vi "Read Path Connection Map.vi"(8 "error in (no error)":errorcluster, 11 "Cal Standard Base in":refnum<class "Cal Standard Base.lvclass">) -> (0 "error out":errorcluster, 2 "Path Connection Map":map{string, string[]}(c390), 3 "Cal Standard Base out":refnum<class "Cal Standard Base.lvclass">)   [LabVIEW 2023, in "RFFixtureCharact.Instruments.lvlib" / "Cal Standard Base.lvclass"]
uses:
  Cal Standard Base.lvclass
  Cal Standard Base.lvclass/Cal Standard Base.ctl
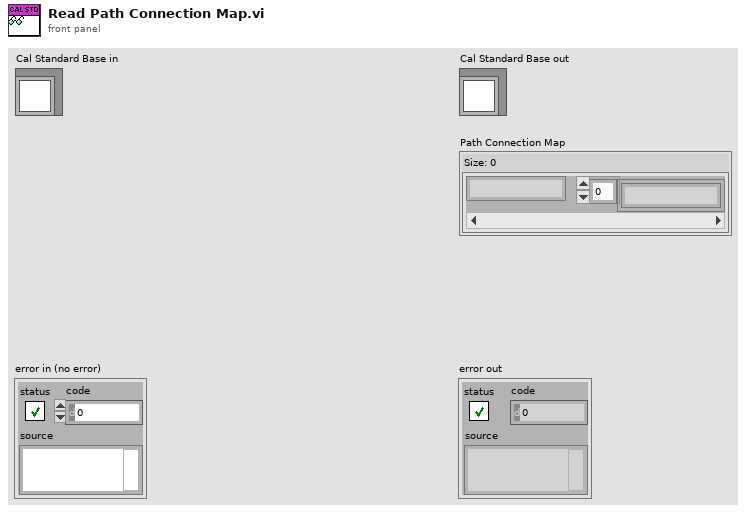
[diagram p1: front panel]
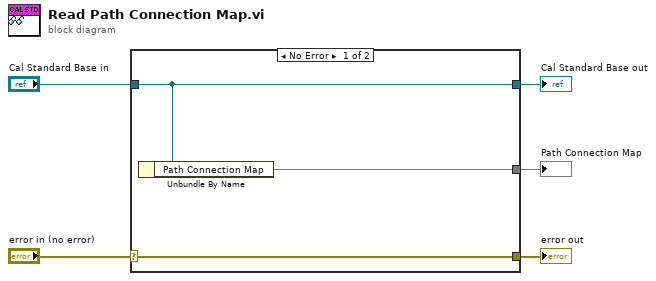
[diagram p0: block diagram]
diagram:
  n1 = case shown="No Error" "error in (no error)" {
    selector: "error in (no error)" -> [w8 w9]
    tunnel: [w8 w9] -> w4
    tunnel: [w7 w10] -> w2
    tunnel: "Cal Standard Base in" -> [w7 w10]
    tunnel: [w6 _] -> w1
    frame No Error {
      n2 = Unbundle By Name(w7) -> ("Path Connection Map"=w6:map{string, string[]})
    }
    frame Error {
    }
  }
  "error out" <- w4
  "Cal Standard Base out" <- w2
  "Path Connection Map" <- w1
